vi "InitMessageMetadata.vi"(9 "ActorLifetime":T1, 10 "ActorRelation":T3, 11 "ActorAlias":string) -> (3 "MessageMetadata":T2 {"AbsoluteTime" format="%<%x %.3X>T"})   [LabVIEW 2020, in "jettl.lvlib"]
uses:
  jettl.lvlib
  ActorLifetime.ctl
  ActorRelation.ctl
  MessageMetadata.ctl
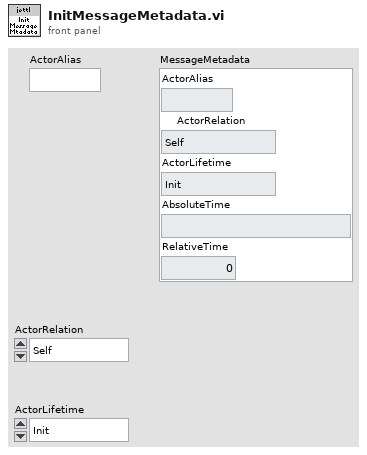
[diagram p1: front panel]
types:
  T1 = typedef "jettl.lvlib/ActorLifetime.ctl" = enum16{"Init", "Spawn", "Setup", "Teardown Before Running", "Running", "Stop Called", "Stopping With Children", "Stopping Without Children", "Teardown After Running", "Stopped"}
  T2 = typedef "jettl.lvlib/MessageMetadata.ctl" = cluster{"ActorAlias":string, "ActorRelation":T3, "ActorLifetime":T1, "AbsoluteTime":timestamp, "RelativeTime":dbl}
  T3 = typedef "jettl.lvlib/ActorRelation.ctl" = enum16{"Self", "Actor"}
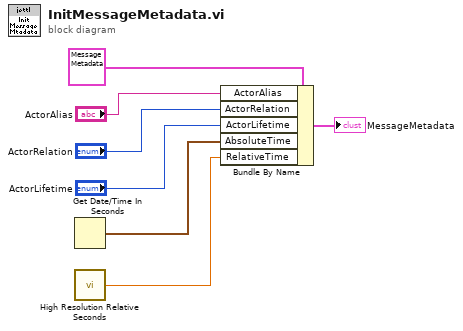
[diagram p0: block diagram]
diagram:
  n1 = Get Date/Time In Seconds() -> (seconds since 1Jan1904=w6:timestamp)
  n2 = call <vilib>:"High Resolution Relative Seconds.vi"() -> ("relative seconds"=w7:dbl)
  n3 = Bundle By Name(cluster=T2 {"ActorAlias"="", "ActorRelation"=enum."Self", "ActorLifetime"=enum."Init", "AbsoluteTime"=timestamp(0 s since 1904-01-01), "RelativeTime"=0.0} ("MessageMetadata"), "ActorAlias"="ActorAlias", "ActorRelation"="ActorRelation", "ActorLifetime"="ActorLifetime", "AbsoluteTime"=w6, "RelativeTime"=w7) -> (→"MessageMetadata":T2)
